vi "SVT UFF58 Read.vi"   [LabVIEW 2017, in "SoundVib_UFF58.lvlib"]
doc: "Reads data from a UFF58 (universal file format) function specified by the <B>function refnum</B> input. This VI also reads the fields in records 1, 2, and 3, returned by ID lines (1-3). You can read a single time domain waveform, a single frequency spectrum, the real and imaginary parts of a frequency spectrum, and any data from a function. The default instance, SVT UFF58 Read Time Waveform, reads a single time domain waveform from a function specified by the <B>function refnum</B> input. Wire data to the <B>function refnum</B> input to determine the polymorphic instance to use or manually select the instance."
uses:
  <vilib>/addons/Sound and Vibration/svt_UFF58/SoundVib_UFF58.lvlib
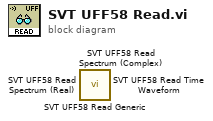
[diagram p0: block diagram]
diagram:
  n1 = call <vilib>:"SVT UFF58 Read Generic.vi"() -> ()  [unwired: 8 in, 8 out]
  n2 = call <vilib>:"SVT UFF58 Read Spectrum (Complex).vi"() -> ()  [unwired: 11 in, 5 out]
  n3 = call <vilib>:"SVT UFF58 Read Spectrum (Real).vi"() -> ()  [unwired: 12 in, 4 out]
  n4 = call <vilib>:"SVT UFF58 Read Time Waveform.vi"() -> ()  [unwired: 12 in, 4 out]
